vi "SetHeadEnable API.vi"(8 "error in (no error)":errorcluster, 9 "Enable":bool, 10 "Head":T1=enum."1", 11 "TopLevel in":refnum<class "TopLevel.lvclass">) -> (0 "error out":errorcluster, 3 "TopLevel out":refnum<class "TopLevel.lvclass">)   [LabVIEW 2022 SP3, in "TopLevel.lvclass"]
uses:
  TopLevel.lvclass
  Typedefs/PrinterHeads--Enum.ctl
  Typedefs/API Command Cluster.ctl
  Typedefs/API Command Enum.ctl
  Common/Controls/HeadHeaterTemperatureEnable--Cluster.ctl
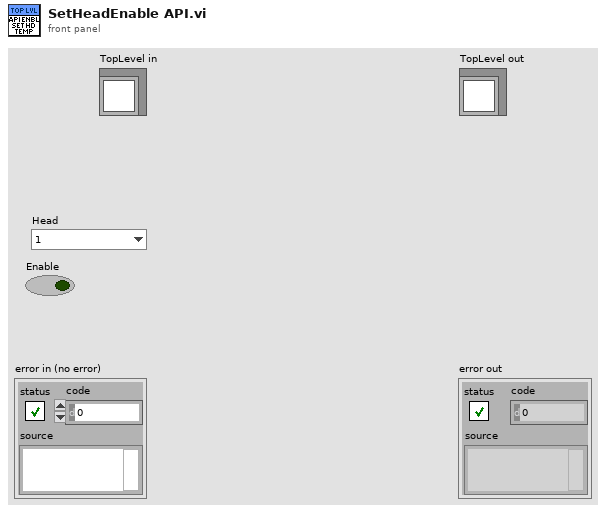
[diagram p1: front panel]
types:
  T1 = typedef "PrinterHeads--Enum.ctl" = enum16{"-1", "1", "2", "3", "4", "5", "6"}
  T2 = typedef "HeadHeaterTemperatureEnable--Cluster.ctl" = cluster{"Head":T1, "Enable":bool}
  T3 = typedef "TopLevel.lvclass/API Command Enum.ctl" = enum16{"Execute Printer Commands", "Pre Purge", "Enable Ink Ch-1", "Enable Ink Ch-2", "Enable Ink Ch-3", "Enable Ink Ch-4", "Enable Ink Ch-5", "Enable Ink Ch-6", "Disable Ink Ch-1", "Disable Ink Ch-2", "Disable Ink Ch-3", "Disable Ink Ch-4", "Disable Ink Ch-5", "Disable Ink Ch-6", "ExecuteIdlePrintCycle", "StopIdlePrintCycle", "Abort", "LoadDLP2GUIConfig", "SaveDLP2GUIConfig", "PrimingMode", "SetHeadTemperature", "EnableHead", "EnableHeadHeat", "SetSystemMode", "HeadPrint", "AbortAll", "Send Printer String"}
  T4 = typedef "TopLevel.lvclass/API Command Cluster.ctl" = cluster{"Command":T3, "Arguments":string, "Data":variant}
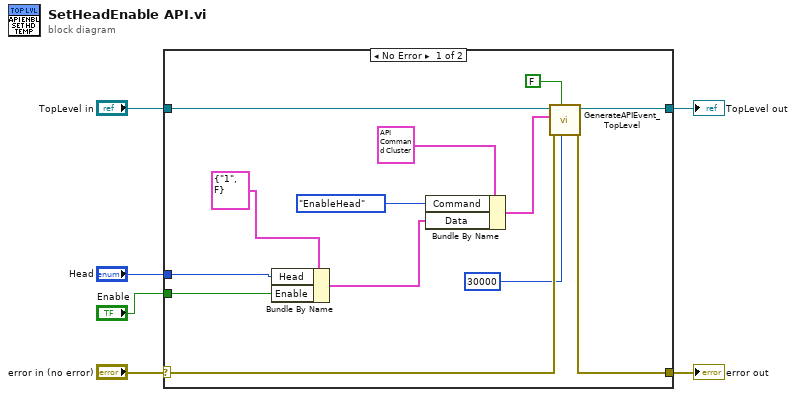
[diagram p0: block diagram]
diagram:
  n1 = case shown="No Error" "error in (no error)" {
    selector: "error in (no error)" -> [w17 w21]
    tunnel: [w16 w21] -> w5
    tunnel: [w19 w20] -> w3
    tunnel: "TopLevel in" -> [w18 w20]
    tunnel: "Head" -> [w9 _]
    tunnel: "Enable" -> [w7 _]
    frame No Error {
      n2 = Bundle By Name(cluster=T2 {"Head"=enum."1", "Enable"=FALSE} ("Cluster"), "Head"=w9, "Enable"=w7) -> (w12:T2)
      n3 = Bundle By Name(cluster=T4 {"Command"=enum."Execute Printer Commands", "Arguments"="", "Data"=variant} ("API Command Cluster"), "Command"=API_Command_Enum."EnableHead", "Data"=w12) -> (w13:T4)
      n4 = call-dynamic "GenerateAPIEvent_TopLevel.vi"("Timeout (ms)"=u32 30000, "Wait (F)"=FALSE, "error in (no error)"=w17, "API Command Cluster"=w13, "TopLevel in"=w18) -> ("error out"=w16:errorcluster, "TopLevel out"=w19:refnum<class "TopLevel.lvclass">)  [unwired: 5 in]
    }
    frame Error {
    }
  }
  "error out" <- w5
  "TopLevel out" <- w3
